vi "Get Configuration Default.vi"(7 "Get Results Default? (F)":bool, 8 "error in (no error)":errorcluster) -> (0 "error out":errorcluster, 3 "Control Default":variant)   [LabVIEW 2020, in "MeasurementLink Measurement Server.lvlib"]
uses:
  MeasurementLink Measurement Server.lvlib
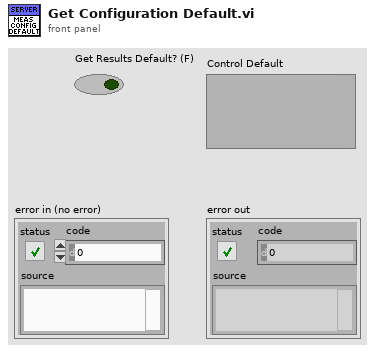
[diagram p1: front panel]
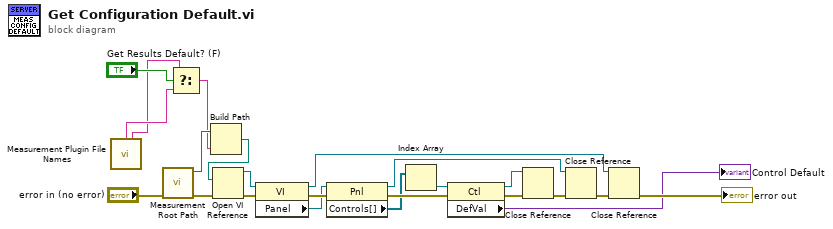
[diagram p0: block diagram]
diagram:
  n1 = call "Measurement Plugin File Names.vi"() -> ("Configuration"=w3:string, "Results"=w1:string)  [unwired: 10 in, 4 out]
  n2 = call "Measurement Root Path.vi"("error in (no error)"="error in (no error)") -> ("error out"=w7:errorcluster, "Measurement Library Path out"=w8:path)  [unwired: 9 in]
  n3 = Select(t=w1, s="Get Results Default? (F)", f=w3) -> (s? t:f=w2:string)
  n4 = Build Path(base path=w8, name or relative path=w2) -> (appended path=w5:path)
  n5 = Open VI Reference(vi path=w5, error in (no error)=w7) -> (vi reference=w11:refnum<vi>, error out=w20:errorcluster)  [unwired: 4 in]
  n6 = property class="VI"(reference=w11, error in=w20) -> (reference out=w16:refnum<vi>, error out=w19:errorcluster, "Panel"=w12:refnum<vi>)
  n7 = property class="Pnl"(reference=w12, error in=w19) -> (reference out=w15:refnum<vi>, error out=w21:errorcluster, "Controls[]"=w13:refnum<vi>[])
  n8 = Index Array(array=w13) -> (element=w22:refnum<vi>)  [unwired: 1 in]
  n9 = property class="Ctl"(reference=w22, error in=w21) -> (reference out=w14:refnum<vi>, error out=w23:errorcluster, "DefVal"=→"Control Default":variant)
  n10 = Close Reference(reference=w14, error in (no error)=w23) -> (error out=w18:errorcluster)
  n11 = Close Reference(reference=w15, error in (no error)=w18) -> (error out=w17:errorcluster)
  n12 = Close Reference(reference=w16, error in (no error)=w17) -> (error out=→"error out":errorcluster)
